vi "Max Read Array.vi"(8 "error in":errorcluster, 11 "Max Pressure Limit in":refnum<class "Pressure Limit.lvclass">) -> (0 "error out":errorcluster, 1 "Changed or First Call?":bool, 2 "Pressure Max SP":dbl[](array[numeric]), 3 "Max Pressure Limit out":refnum<class "Pressure Limit.lvclass">)   [LabVIEW 2023, in "Pressure Limit.lvclass"]
uses:
  Pressure Limit.lvclass
  Parents/Limit/Limit.lvclass
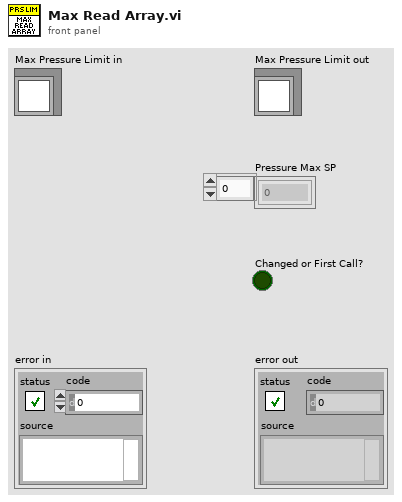
[diagram p1: front panel]
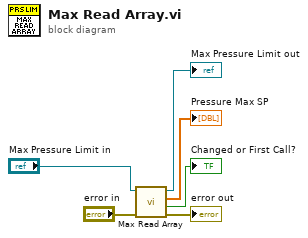
[diagram p0: block diagram]
diagram:
  n1 = call-parent "Max Read Array.vi"("error in"="error in", "Max Limit in"="Max Pressure Limit in") -> ("error out"=→"error out":errorcluster, "Changed or First Call?"=→"Changed or First Call?":bool, "Current Max SP"=→"Pressure Max SP":dbl[], "Max Limit out"=→"Max Pressure Limit out":refnum<class "Pressure Limit.lvclass">)  [unwired: 6 in]
